vi "myRIO_BRig_RT_dataExp_Tcycle_Timeout.vi"() -> (2 "output_Tcycle_Timeout":i32)   [LabVIEW 2014]
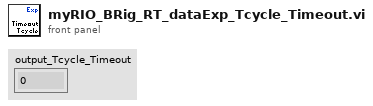
[diagram p1: front panel]
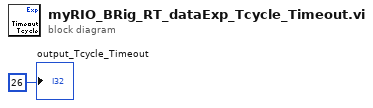
[diagram p0: block diagram]
diagram:
  "output_Tcycle_Timeout" <- 26 ("output_iBlock")
